vi "tor_switch.vi"() -> ()   [LabVIEW 2025]
panel:
  out "SENSx":bool
  in  "IN1":bool
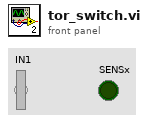
[diagram p1: front panel]
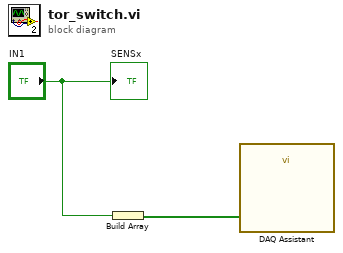
[diagram p0: block diagram]
diagram:
  n1 = Build Array("IN1") -> (w2:bool[])
  n2 = call "DAQ Assistant"("data"=w2) -> ()  [unwired: 17 in, 2 out]
  "SENSx" <- "IN1"
